vi "LASER_EnableColors.vi"(8 "error in":errorcluster, 10 "Enabled Colors":bool[](array[boolean]), 11 "Constant Output Configuration":T1) -> (0 "error out":errorcluster, 3 "Constant Output Configuration (dup)":T1)   [LabVIEW 2010]
uses:
  <vilib>/DAQmx/write.llb/DAQmx Write (Digital 1D Bool NChan 1Samp 1Line).vi
  <vilib>/DAQmx/write.llb/DAQmx Write (Analog 1D DBL NChan 1Samp).vi
  <vilib>/daqmx/miscellaneous.llb/DAQmx Fill In Error Info.vi
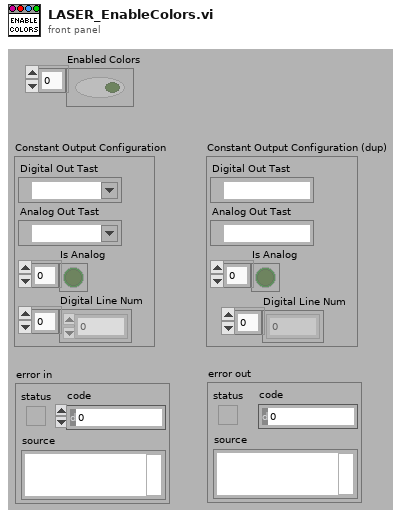
[diagram p1: front panel]
types:
  T1 = cluster{"Digital Out Tast":refnum<k21>, "Analog Out Tast":refnum<k21>, "Is Analog":bool[], "Digital Line Num":u32[]}
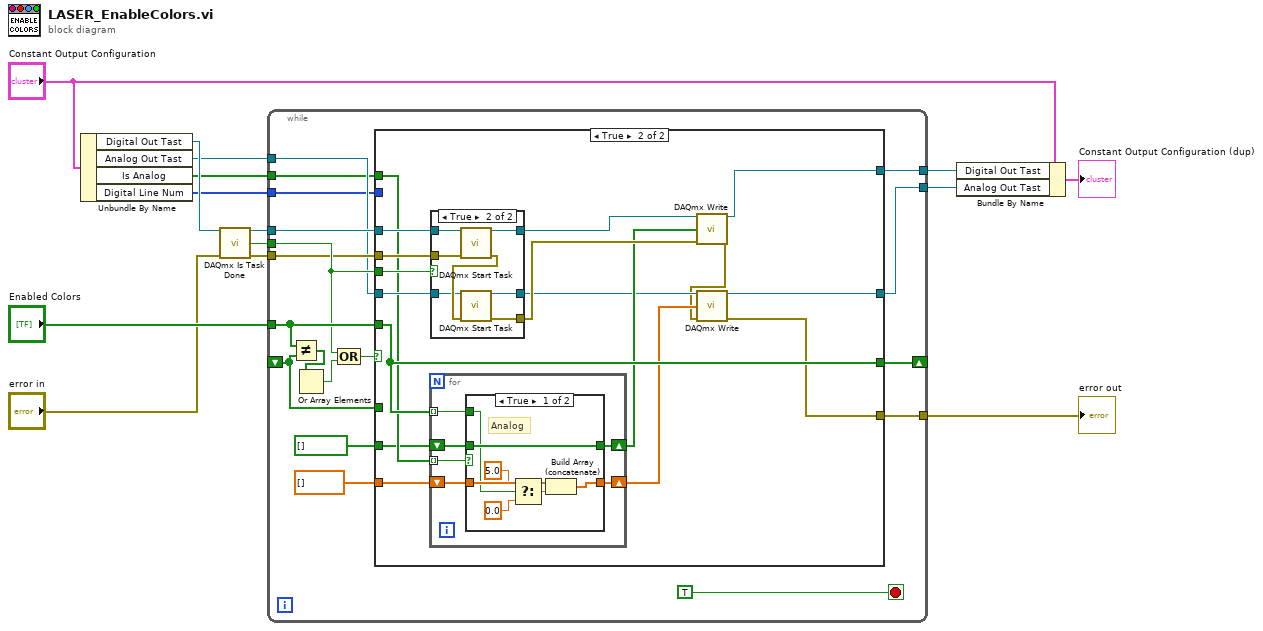
[diagram p0: block diagram]
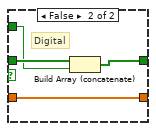
[diagram p3: hidden frame]
diagram:
  n1 = Unbundle By Name("Constant Output Configuration") -> ("Digital Out Tast"=w12:refnum<k21>, "Analog Out Tast"=w8:refnum<k21>, "Is Analog"=w4:bool[], "Digital Line Num"=w3:u32[])
  n2 = call <vilib>:"DAQmx Is Task Done.vi"("task/channels in"=w12, "error in"="error in") -> ("task out"=w9:refnum<k21>, "task done?"=w10:bool, "error out"=w6:errorcluster)  [unwired: 11 in]
  n3 = while {
    tunnel: "Enabled Colors" -> [w26]
    shift-right: [w27] -> _
    shift-left: _ -> [w28]
    tunnel: w10 -> [w25]
    tunnel: w9 -> [w23]
    tunnel: w8 -> [w22]
    tunnel: w6 -> [w24]
    tunnel: [w21] -> w5
    tunnel: w4 -> [w20]
    tunnel: w3 -> [w19]
    tunnel: [w16] -> w2
    tunnel: [w15] -> w1
    stop <- TRUE stop-if-true
    n4 = Not Equal?(x=w26, y=w28) -> (x != y?=w31:bool[])
    n5 = Or Array Elements(Boolean array=w31) -> (logical OR=w30:bool)
    n6 = Compound Arithmetic op=OR(w25, w30) -> (w29:bool)
    n7 = case shown="True" w29 {
      tunnel: w28 -> [w36 _]
      tunnel: [w36 w49] -> w27
      tunnel: w26 -> [_ w49]
      tunnel: w25 -> [_ w53]
      tunnel: w24 -> [w35 w52]
      tunnel: w23 -> [w33 w51]
      tunnel: w22 -> [w34 w50]
      tunnel: [w35 w37] -> w21
      tunnel: w20 -> [_ w48]
      tunnel: w19 -> [_ _]
      tunnel: bool[] [] ("array") -> [_ w47]
      tunnel: dbl[] [] ("array") -> [_ w46]
      tunnel: [w33 w41] -> w16
      tunnel: [w34 w38] -> w15
      frame False {
      }
      frame True {
        n8 = for {
          tunnel: w49 -> [w54] mode=indexing
          tunnel: w48 -> [w59] mode=indexing
          shift-right: [w56] -> w40
          shift-left: w46 -> [w57]
          shift-right: [w55] -> w43
          shift-left: w47 -> [w58]
          n9 = case shown="True" w59 {
            tunnel: w58 -> [w64 w70]
            tunnel: w57 -> [w66 w68]
            tunnel: [w65 w68] -> w56
            tunnel: [w64 w69] -> w55
            tunnel: w54 -> [w63 w67]
            frame True {
              # "Analog"
              n10 = Select(t=5.0, s=w63, f=0.0) -> (s? t:f=w62:dbl)
              n11 = Build Array (concatenate)(w66, w62) -> (w65:dbl[])
            }
            frame False {
              # "Digital"
              n12 = Build Array (concatenate)(w70, w67) -> (w69:bool[])
            }
          }
        }
        n13 = case shown="True" w53 {
          tunnel: w52 -> [w71 w80]
          tunnel: w51 -> [w72 w79]
          tunnel: w50 -> [w73 w77]
          tunnel: [w73 w75] -> w42
          tunnel: [w72 w76] -> w45
          tunnel: [w71 w74] -> w44
          frame False {
          }
          frame True {
            n14 = call <vilib>:"DAQmx Start Task.vi"("task/channels in"=w79, "error in"=w80) -> ("task out"=w76:refnum<k21>, "error out"=w78:errorcluster)  [unwired: 12 in]
            n15 = call <vilib>:"DAQmx Start Task.vi"("task/channels in"=w77, "error in"=w78) -> ("task out"=w75:refnum<k21>, "error out"=w74:errorcluster)  [unwired: 12 in]
          }
        }
        n16 = call-poly <vilib>:"DAQmx Write.vi"("task/channels in"=w45, "data"=w43, "error in"=w44) -> ("task out"=w41:refnum<k21>, "error out"=w39:errorcluster)  [unwired: 10 in, 1 out]
        n17 = call-poly <vilib>:"DAQmx Write.vi"("task/channels in"=w42, "data"=w40, "error in"=w39) -> ("task out"=w38:refnum<k21>, "error out"=w37:errorcluster)  [unwired: 10 in, 1 out]
      }
    }
  }
  "error out" <- w5
  n18 = Bundle By Name(cluster="Constant Output Configuration", "Digital Out Tast"=w2, "Analog Out Tast"=w1) -> (→"Constant Output Configuration (dup)":T1)
